vi "PLC Unit Test.vi"() -> ()   [LabVIEW 2018]
uses:
  PPLs/PLC/Light Stack/Light Stack.lvlibp/Custom Controls/Light Select.ctl
  PPLs/PLC/Light Stack/Light Stack.lvlibp/Custom Controls/Light Mode.ctl
  PPLs/PLC/Parent/PLC.lvlibp/PLC.lvclass
  PPLs/PLC/Light Stack/Light Stack.lvlibp
panel:
  in  "Device Name":string="PLC-1"
  in  "PPLs Folder Path":path
  in  "INI File Path":path
  in  "State":T1
  in  "Light Select":T2
  in  "stop":bool
  out "Analog In":dbl[](array[numeric])
  in  "Analog out":dbl[](array[numeric])
  out "Digital In":bool[](array[boolean])
  in  "Digital Out":bool[](array[boolean])
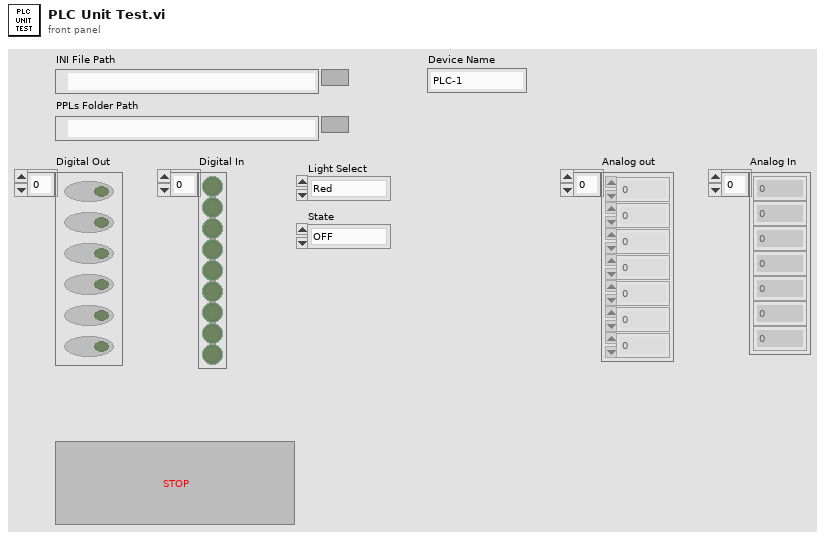
[diagram p1: front panel]
types:
  T1 = typedef "Light Stack.lvlibp/Light Mode.ctl" = enum16{"OFF", "ON", "BLINK"}
  T2 = typedef "Light Stack.lvlibp/Light Select.ctl" = enum16{"Red", "Amber", "Green", "Blue"}
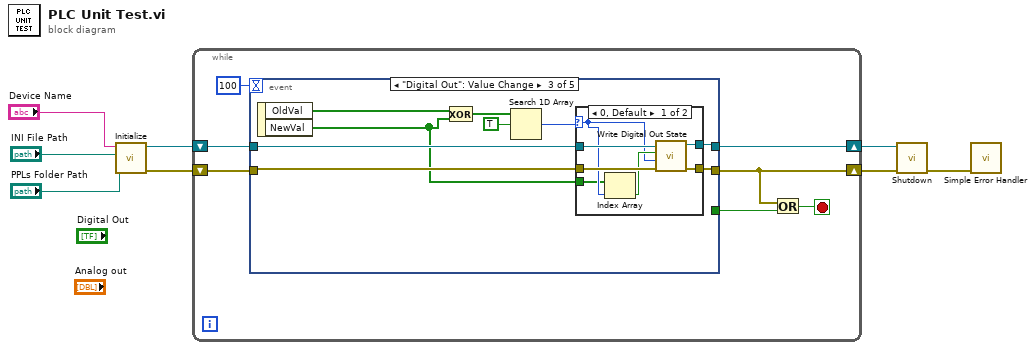
[diagram p0: block diagram]
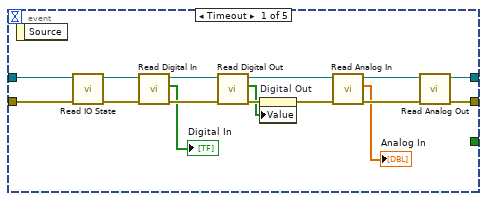
[diagram p2: hidden frame]
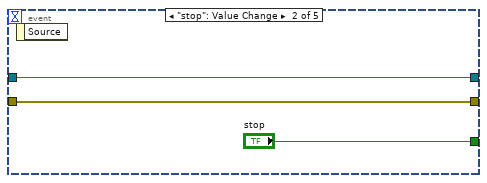
[diagram p3: hidden frame]
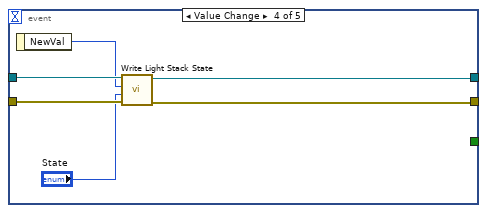
[diagram p5: hidden frame]
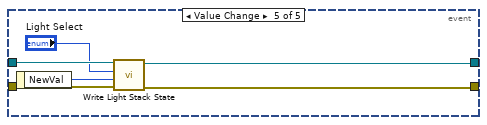
[diagram p6: hidden frame]
diagram:
  n1 = call "Initialize.vi"("PPLs Folder Path"="PPLs Folder Path", "INI File Path"="INI File Path", "Device"="Device Name") -> ("error out"=w7:errorcluster, "PLC out"=w8:refnum<class "PLC.lvclass">)  [unwired: 7 in]
  n2 = while {
    shift-right: [w12] -> w6
    shift-left: w8 -> [w14]
    shift-right: [w11] -> w5
    shift-left: w7 -> [w13]
    stop <- w10 stop-if-true
    n3 = event shown="[2] \"Digital Out\": Value Change" {
      selector: _ -> [_ _ _ _ _]
      dyn-events: _ -> [_ _ _ _ _]
      timeout: 100 -> [_ _ _ _ _]
      tunnel: w14 -> [w18 w34 w40 w58 w64]
      tunnel: w13 -> [w19 w33 w43 w57 w60]
      tunnel: [w29 w33 w42 w55 w59] -> w11
      tunnel: [w28 w34 w41 w56 w63] -> w12
      tunnel: [_ "stop" _ _ _] -> w9
      event Timeout {
        n4 = event-data() -> ()  [unwired: 1 in, 1 out]
        n5 = call "Read IO State.vi"("error in"=w19, "PLC in"=w18) -> ("error out"=w16:errorcluster, "PLC out"=w17:refnum<class "PLC.lvclass">)  [unwired: 8 in]
        n6 = call "Read Digital In.vi"("error in"=w16, "PLC in"=w17) -> ("error out"=w31:errorcluster, "Digital In"=→"Digital In":bool[], "PLC out"=w27:refnum<class "PLC.lvclass">)  [unwired: 7 in]
        n7 = call "Read Digital Out.vi"("error in"=w31, "PLC in"=w27) -> ("error out"=w22:errorcluster, "Digital Out"=w20:bool[], "PLC out"=w26:refnum<class "PLC.lvclass">)  [unwired: 7 in]
        n8 = property on="Digital Out" class="Arr (strict)"(error in=w22, "Value"=w20) -> (error out=w21:errorcluster)  [unwired: 1 in, 1 out]
        n9 = call "Read Analog In.vi"("error in"=w21, "PLC in"=w26) -> ("error out"=w30:errorcluster, "Analog In"=→"Analog In":dbl[], "PLC out"=w25:refnum<class "PLC.lvclass">)  [unwired: 7 in]
        n10 = call "Read Analog Out.vi"("error in"=w30, "PLC in"=w25) -> ("error out"=w29:errorcluster, "PLC out"=w28:refnum<class "PLC.lvclass">)  [unwired: 7 in, 1 out]
      }
      event "stop": Value Change {
        n11 = event-data() -> ()  [unwired: 1 in, 1 out]
      }
      event "Digital Out": Value Change {
        n12 = event-data() -> ("OldVal"=w39:bool[], "NewVal"=w35:bool[])  [unwired: 1 in]
        n13 = Exclusive Or(1:w35, 2:w39) -> (0:w37:bool[])
        n14 = Search 1D Array(1D array=w37, element=TRUE) -> (index of element=w36:i32)  [unwired: 1 in]
        n15 = case shown="0, Default" w36 {
          selector: w36 -> [w45 _]
          tunnel: w43 -> [w50 w51]
          tunnel: [w49 w51] -> w42
          tunnel: [w48 w52] -> w41
          tunnel: w40 -> [w47 w52]
          tunnel: w35 -> [w44 _]
          frame 0, Default {
            n16 = Index Array(array=w44, index=w45) -> (element=w46:bool)
            n17 = call "Write Digital Out State.vi"("error in"=w50, "Selection"=w45, "Value"=w46, "PLC in"=w47) -> ("error out"=w49:errorcluster, "PLC out"=w48:refnum<class "PLC.lvclass">)  [unwired: 6 in]
          }
          frame -1 {
          }
        }
      }
      event Value Change {
        n18 = event-data() -> ("NewVal"=w54:T2)  [unwired: 1 in]
        n19 = call "Write Light Stack State.vi"("error in"=w57, "State"="State", "Light Select"=w54, "PLC in"=w58) -> ("error out"=w55:errorcluster, "PLC out"=w56:refnum<class "PLC.lvclass">)  [unwired: 6 in]
      }
      event Value Change {
        n20 = event-data() -> ("NewVal"=w61:T1)  [unwired: 1 in]
        n21 = call "Write Light Stack State.vi"("error in"=w60, "State"=w61, "Light Select"="Light Select", "PLC in"=w64) -> ("error out"=w59:errorcluster, "PLC out"=w63:refnum<class "PLC.lvclass">)  [unwired: 6 in]
      }
    }
    n22 = Or(x=w11, y=w9) -> (x .or. y?=w10:bool)
  }
  n23 = call "Shutdown.vi"("error in"=w5, "PLC in"=w6) -> ("error out"=w4:errorcluster)  [unwired: 8 in, 1 out]
  n24 = call <vilib>:"Simple Error Handler.vi"("error in (no error)"=w4) -> ()  [unwired: 4 in, 5 out]
